vi "NI-Switch Initialization VI.vi"(8 "error in (no error)":errorcluster, 10 "Custom XML":string, 11 "Device Item Ref in":T2 format="%.0x") -> (0 "error out":errorcluster, 3 "Device Item Ref out":T2 format="%.0x")   [LabVIEW 2011, in "NI-Switch Relay Custom Device.lvlib"]
uses:
  NI-Switch Relay Custom Device.lvlib
  <vilib>/NI Veristand/Custom Device API/Custom Device Item Ref.ctl
  <instrlib>/niSwitch/niSwitch.LLB/niSwitch Topologies.ctl
  <vilib>/NI Veristand/Custom Device API/Custom Device API.lvlib
panel:
  in  "Rate Decimation":i32=1
  in  "Cancel Button":bool
  in  "OK Button":bool
  in  "Number of Desired Relays":i32
  in  "topology name":T1="1127/2-Wire 32x1 Mux" caption="Topology Name"
  out "Avaliable Relays":string[](array[string])
  out "Max. number of relays\n for the selected topology:":i32
  in  "Resource Name":string
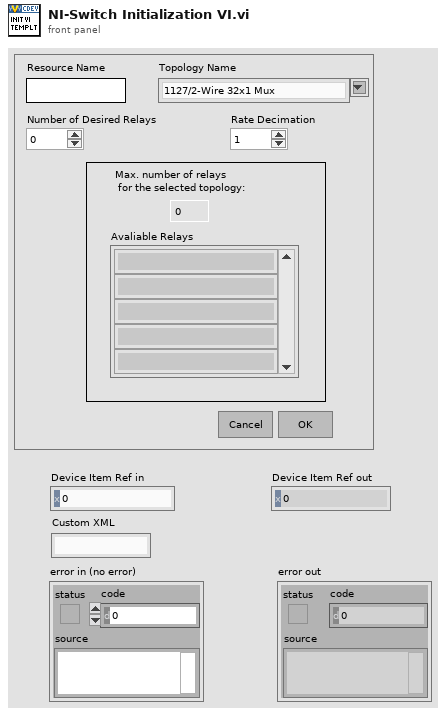
[diagram p1: front panel]
types:
  T1 = typedef "niSwitch Topologies.ctl" = string
  T2 = typedef "Custom Device API.lvlib/Custom Device Item Ref.ctl" = u64
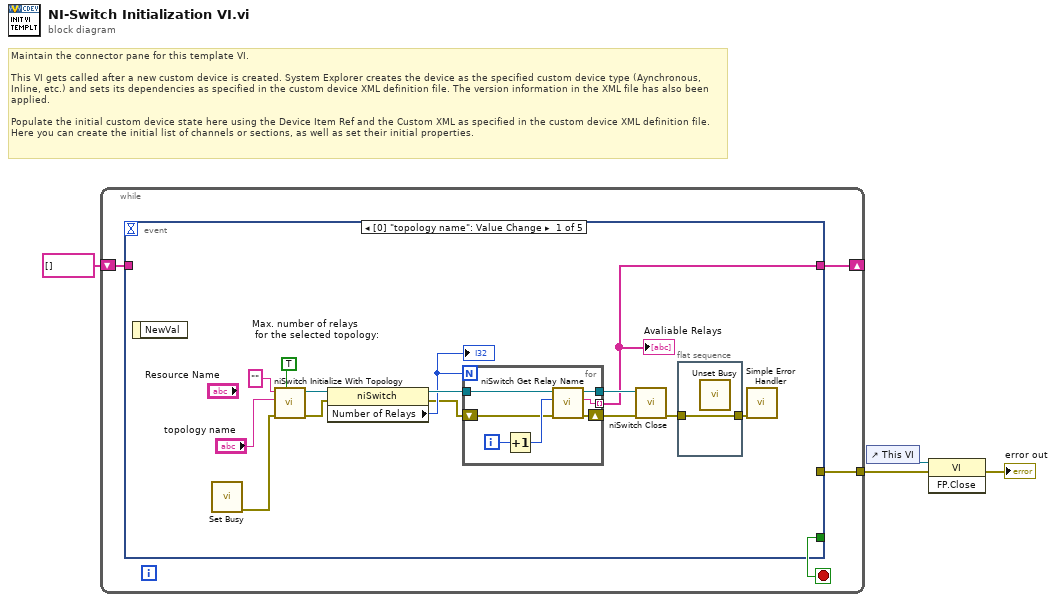
[diagram p0: block diagram]
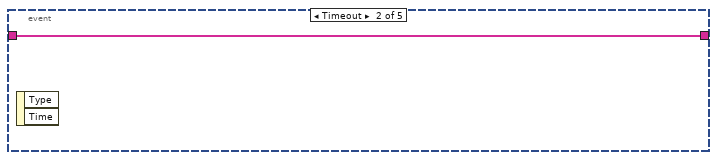
[diagram p2: hidden frame]
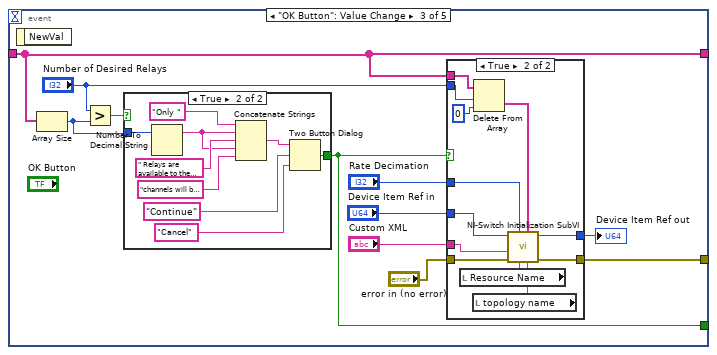
[diagram p3: hidden frame]
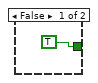
[diagram p4: hidden frame]
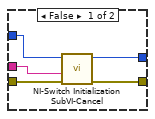
[diagram p5: hidden frame]
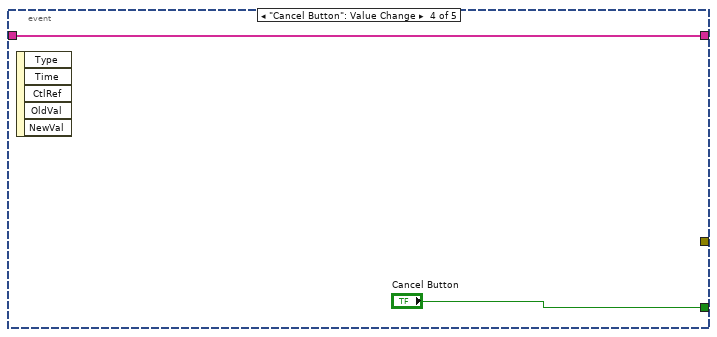
[diagram p6: hidden frame]
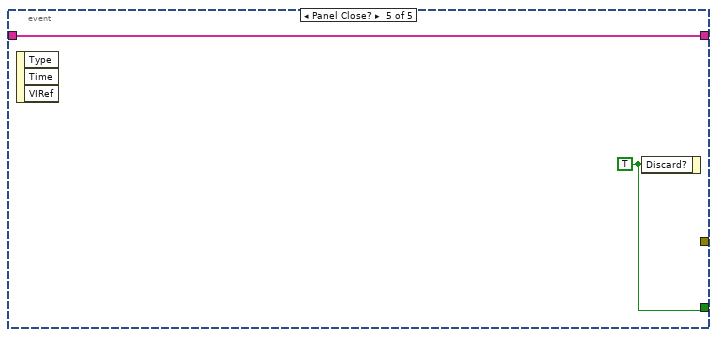
[diagram p7: hidden frame]
diagram:
  # "Maintain the connector pane for this template VI.\n\nThis VI gets called after a new custom device is created. System Explorer creates the device as the specified custom device type (Aynchronous, Inline, etc.) and sets its dependencies as specified in the custom device XML definition file. The version information in the XML file has also been applied.\n\nPopulate the initial custom device state here using the Device Item Ref and the Custom XML as specified in the custom device XML definition file. Here you can create the initial list of channels or sections, as well as set their initial properties."
  n1 = while {
    shift-right: [w7] -> _
    shift-left: string[] [] -> [w6]
    tunnel: [w5] -> w2
    stop <- w8 stop-if-true
    n2 = event shown="[0] \"topology name\": Value Change" {
      selector: _ -> [_ _ _ _ _]
      dyn-events: _ -> [_ _ _ _ _]
      timeout: _ -> [_ _ _ _ _]
      tunnel: [_ _ w40 "Cancel Button" w72] -> w8
      tunnel: [w13 w31 w38 w70 w73] -> w7
      tunnel: w6 -> [_ w31 w38 w70 w73]
      tunnel: [_ _ w37 _ _] -> w5
      event Value Change {
        n3 = event-data() -> ()  [unwired: 1 in, 1 out]
        n4 = call <vilib>:"Set Busy.vi"() -> ("error out"=w12:errorcluster)  [unwired: 10 in, 1 out]
        n5 = call <instrlib>:"niSwitch Initialize With Topology.vi"("simulate (boolean value)"=TRUE, "error in (no error)"=w12, "topology name"="topology name", "resource name"="") -> ("error out"=w17:errorcluster, "instrument handle out"=w16:refnum<k15>)  [unwired: 6 in]
        n6 = property class="niSwitch"(reference=w16, error in=w17) -> (reference out=w20:refnum<k15>, error out=w18:errorcluster, "Number of Relays"=w19:i32)
        "Max. number of relays\n for the selected topology:" <- w19
        n7 = for {
          N: w19 -> [_]
          tunnel: w20 -> [w25]
          tunnel: [w29] -> w13 mode=indexing
          tunnel: [w27] -> w22
          shift-right: [w26] -> w21
          shift-left: w18 -> [w24]
          i -> [w30]
          n8 = Increment(x=w30) -> (x+1=w28:i32)
          n9 = call <instrlib>:"niSwitch Get Relay Name.vi"("error in (no error)"=w24, "index (1)"=w28, "instrument handle"=w25) -> ("error out"=w26:errorcluster, "relay name"=w29:string, "instrument handle out"=w27:refnum<k15>)  [unwired: 6 in]
        }
        "Avaliable Relays" <- w13
        n10 = call <instrlib>:"niSwitch Close.vi"("error in (no error)"=w21, "instrument handle"=w22) -> ("error out"=w10:errorcluster)  [unwired: 9 in]
        n11 = flat-sequence {
          tunnel: [w23] -> w11
          tunnel: w10 -> [w23]
          frame #0 {
            n12 = call <vilib>:"Unset Busy.vi"() -> ()  [unwired: 11 in, 1 out]
          }
        }
        n13 = call <vilib>:"Simple Error Handler.vi"("error in (no error)"=w11) -> ()  [unwired: 4 in, 5 out]
      }
      event Timeout {
        n14 = event-data() -> ()  [unwired: 1 in, 2 out]
      }
      event "OK Button": Value Change {
        n15 = event-data() -> ()  [unwired: 1 in, 1 out]
        n16 = Array Size(array=w38) -> (size(s)=w42:i32)
        n17 = Greater?(x="Number of Desired Relays", y=w42) -> (0:w41:bool)
        n18 = case shown="True" w41 {
          tunnel: w42 -> [_ w51]
          tunnel: [TRUE ("T button?") w49] -> w40
          frame False {
          }
          frame True {
            n19 = Number To Decimal String(number=w51) -> (decimal integer string=w47:string)  [unwired: 1 in]
            n20 = Concatenate Strings("Only " ("message"), w47, " Relays are available to the selected topology.\nWould you like to continue?\nIf you continue only " ("string"), w47, "channels will be created." ("string")) -> (w50:string)
            n21 = Two Button Dialog(message=w50, 1:"Cancel" ("T button name (\"OK\")"), 2:"Continue" ("T button name (\"OK\")")) -> (T button?=w49:bool)
          }
        }
        n22 = case shown="True" w40 {
          tunnel: "Number of Desired Relays" -> [_ w69]
          tunnel: w38 -> [_ w67]
          tunnel: [w56 w63] -> w37
          tunnel: "error in (no error)" -> [w57 w62]
          tunnel: "Rate Decimation" -> [_ w61]
          tunnel: "Device Item Ref in" -> [w54 w60]
          tunnel: "Custom XML" -> [w53 w59]
          tunnel: [w55 w58] -> w32
          frame False {
            n23 = call "NI-Switch Initialization SubVI-Cancel.vi"("error in (no error)"=w57, "Custom XML"=w53, "Device Item Ref in"=w54) -> ("error out"=w56:errorcluster, "Device Item Ref out"=w55:T2)  [unwired: 7 in]
          }
          frame True {
            n24 = local read "Resource Name"() -> (w65:string)
            n25 = local read "topology name"() -> (w64:T1)
            n26 = Delete From Array(array=w67, length=w69, index=0) -> (deleted portion=w66:string[])  [unwired: 1 out]
            n27 = call "NI-Switch Initialization SubVI.vi"("Topology Name"=w64, "Channels Array"=w66, "Resource Name"=w65, "Decimation"=w61, "error in (no error)"=w62, "Custom XML"=w59, "Device Item Ref in"=w60) -> ("error out"=w63:errorcluster, "Device Item Ref out"=w58:T2)  [unwired: 3 in]
          }
        }
        "Device Item Ref out" <- w32
      }
      event "Cancel Button": Value Change {
        n28 = event-data() -> ()  [unwired: 1 in, 5 out]
      }
      event Panel Close? {
        w72 = TRUE ("Discard?")
        n29 = event-data() -> ()  [unwired: 1 in, 3 out]
        n30 = event-data("Discard?"=w72) -> ()  [unwired: 1 in, 1 out]
      }
    }
  }
  n31 = control-ref of="This VI"() -> (w3:refnum<vi>)
  n32 = invoke class="VI" method="FP.Close"(reference=w3, error in=w2) -> (error out=→"error out":errorcluster)  [unwired: 1 in, 2 out]
